vi "Wizard Global.vi"() -> ()   [LabVIEW 2021]
panel:
  in  "Error dialog":string="Reinstall the NI LabVIEW %s Toolkit. If this error persists, contact National Instruments for technical support."
  in  "Choice2":string="Directly choose a sample project\nChoose from all sample projects and create a network communication system based on the sample project that you choose.\n"
  in  "Choice1":string="Follow step-by-step instructions to choose a sample project\nSpecify the properties for your network communication system, choose from recommended sample projects, and create a network communication system."
  in  "Start Question":string="How do you want to create %s %s network communication system?"
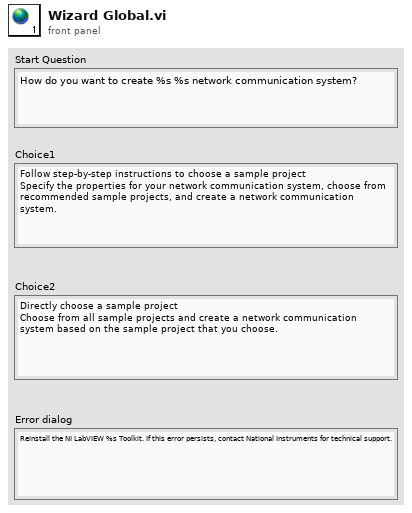
[diagram p1: front panel]
diagram:
